vi "Color Sensor V3 Read8.vi"(8 "error in (no error)":errorcluster, 10 "Registers":T4, 11 "ColorSensorDevRef":T1={"I2CDevRef"={"DevStatus"={"status"=FALSE, "code"=0, "source"=""}, "Device Address"=0, "Handle"=0, "I2C Bus"=enum."Invalid"}} {"I2CDevRef"."Device Address" format="%.0x"}) -> (0 "error out":errorcluster, 2 "Data":u8, 3 "ColorSensorDevRef out":T1={"I2CDevRef"={"DevStatus"={"status"=FALSE, "code"=0, "source"=""}, "Device Address"=0, "Handle"=0, "I2C Bus"=enum."Invalid"}} {"I2CDevRef"."Device Address" format="%.0x"})   [LabVIEW 2023]
uses:
  Typedef/Color Sensor V3 DevRef.ctl
  <vilib>/Rock Robotics/WPI/I2C/WPI_I2CDevRef.ctl
  <vilib>/Rock Robotics/SystemInterfaces/i2clib/i2c_bus.ctl
  Typedef/Color Sensor V3 Registers.ctl
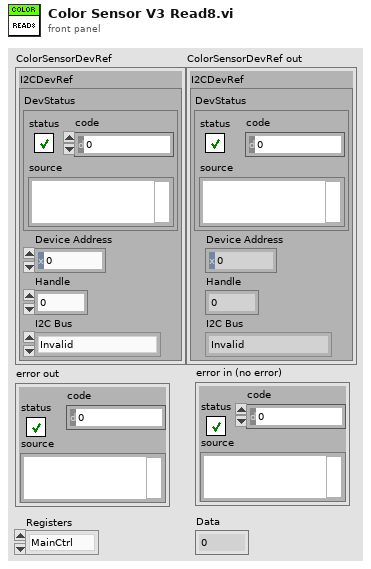
[diagram p1: front panel]
types:
  T1 = typedef "Color Sensor V3 DevRef.ctl" = cluster{"I2CDevRef":T2}
  T2 = typedef "WPI_I2CDevRef.ctl" = cluster{"DevStatus":errorcluster, "Device Address":u8, "Handle":i32, "I2C Bus":T3}
  T3 = typedef "i2c_bus.ctl" = enum16{"I2C On-Board", "I2C MXP", "Invalid"}
  T4 = typedef "Color Sensor V3 Registers.ctl" = enum16{"MainCtrl", "ProximitSensorLED", "ProximitySensorPulse", "ProximitySensorRate", "LightSensorMeasurementRate", "LightSensorGainRegister", "PartIDRegister", "MainStatus", "ProximityData", "ProximityData1", "InfraredData", "InfraredData1", "InfraredData2", "GreenData", "GreenData1", "GreenData2", "BlueData", "BlueData1", "BlueData2", "RedData", "RedData1", "RedData2"}
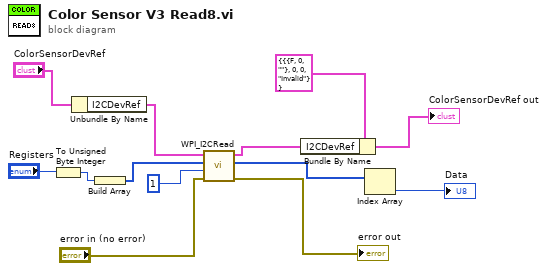
[diagram p0: block diagram]
diagram:
  n1 = To Unsigned Byte Integer(number="Registers") -> (unsigned 8bit integer=w10:u8)
  n2 = Unbundle By Name("ColorSensorDevRef") -> ("I2CDevRef"=w12:T2)
  n3 = Build Array(w10) -> (w9:u8[])
  n4 = call <vilib>:"WPI_I2CRead.vi"("error in (no error)"="error in (no error)", "I2CBytesToRead"=u8 1, "I2CRegister"=w9, "I2CDevRef"=w12) -> ("error out"=→"error out":errorcluster, "Data Out"=w2:u8[], "I2CDevRef"=w5:T2)  [unwired: 5 in]
  n5 = Bundle By Name(cluster=T1 {"I2CDevRef"={"DevStatus"={"status"=FALSE, "code"=0, "source"=""}, "Device Address"=0, "Handle"=0, "I2C Bus"=enum."Invalid"}} ("ColorSensorDevRef"), "I2CDevRef"=w5) -> (→"ColorSensorDevRef out":T1)
  n6 = Index Array(array=w2) -> (element=→"Data":u8)  [unwired: 1 in]
